vi "PathPlanner_PathConstraints_Test.vi"(8 "error in (no error)":errorcluster) -> (0 "error out":errorcluster, 3 "All Passed":bool)   [LabVIEW 2019]
uses:
  <vilib>/Rock Robotics/WPI/ThirdParty/JAS_Junk/TrajLib/Trajectory_Library.lvlib
  <vilib>/Rock Robotics/WPI/ThirdParty/MJansen/PathPlanner/PathPlanner24.lvlib
panel:
  out "Passed 2":bool
  out "Passed 1":bool
  # "Getters"
  # "JSON Parse"
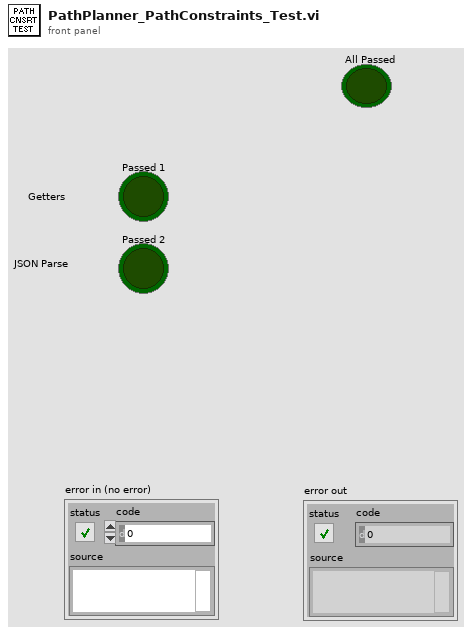
[diagram p1: front panel]
types:
  T1 = typedef "PathPlanner24.lvlib/PathPlannerPathConstraints.ctl" = cluster{"MaxVelocityMps;":dbl, "MaxAccelerationMpsSq;":dbl, "MaxAngularVelRadPsEc;":dbl, "MaxAngularAccRadPSecSq":dbl, "Exists":bool}
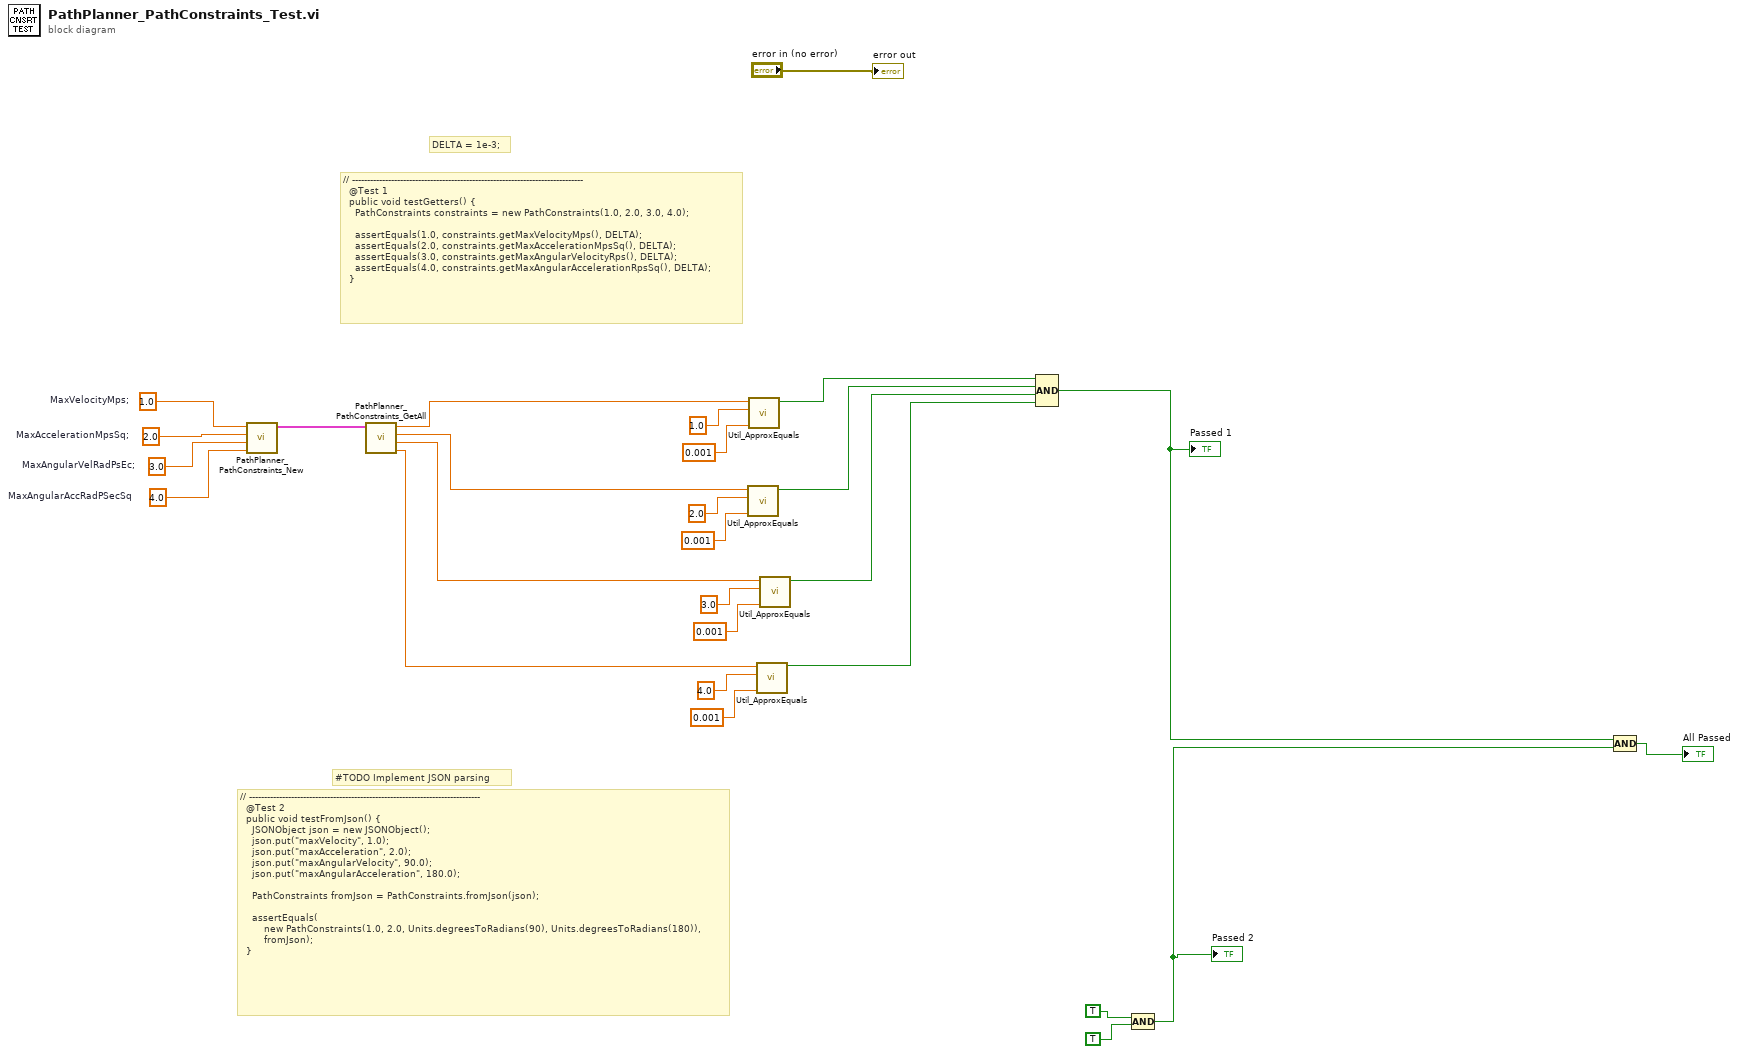
[diagram p0: block diagram]
diagram:
  w20 = 1.0  # MaxVelocityMps;
  w21 = 2.0  # MaxAccelerationMpsSq;
  w22 = 3.0  # MaxAngularVelRadPsEc;
  w23 = 4.0  # MaxAngularAccRadPSecSq
  # "#TODO Implement JSON parsing"
  # "// -----------------------------------------------------------------------------\n  @Test 2\n  public void testFromJson() {\n    JSONObject json = new JSONObject();\n    json.put(\"maxVelocity\", 1.0);\n    json.put(\"maxAcceleration\", 2.0);\n    json.put(\"maxAngularVelocity\", 90.0);\n    json.put(\"maxAngularAcceleration\", 180.0);\n\n    PathConstraints fromJson = PathConstraints.fromJson(json);\n\n    assertEquals(\n        new PathConstraints(1.0, 2.0, Units.degreesToRadians(90), Units.degreesToRadians(180)),\n        fromJson);\n  }"
  # "// -----------------------------------------------------------------------------\n  @Test 1\n  public void testGetters() {\n    PathConstraints constraints = new PathConstraints(1.0, 2.0, 3.0, 4.0);\n\n    assertEquals(1.0, constraints.getMaxVelocityMps(), DELTA);\n    assertEquals(2.0, constraints.getMaxAccelerationMpsSq(), DELTA);\n    assertEquals(3.0, constraints.getMaxAngularVelocityRps(), DELTA);\n    assertEquals(4.0, constraints.getMaxAngularAccelerationRpsSq(), DELTA);\n  }"
  # "DELTA = 1e-3;"
  n1 = call <vilib>:"PathPlanner_PathConstraints_New.vi"("MaxAngularAccRadPSecSq"=w23, "MaxAngularVelRadPsEc;"=w22, "MaxAccelerationMpsSq;"=w21, "MaxVelocityMps;"=w20) -> ("PathPlannerConstraints"=w14:T1)  [unwired: 7 in]
  n2 = call <vilib>:"PathPlanner_PathConstraints_GetAll.vi"("PathPlannerConstraints"=w14) -> ("MaxAngularAccRadPSecSq"=w6:dbl, "MaxAngularVelRadPsEc;"=w7:dbl, "MaxAccelerationMpsSq;"=w8:dbl, "MaxVelocityMps;"=w9:dbl)  [unwired: 7 in]
  n3 = call <vilib>:"Util_ApproxEquals.vi"("Tolerance"=0.001, "Value 2"=2.0, "Value 1"=w8) -> ("ApproxEquals"=w15:bool)  [unwired: 8 in]
  n4 = call <vilib>:"Util_ApproxEquals.vi"("Tolerance"=0.001, "Value 2"=1.0, "Value 1"=w9) -> ("ApproxEquals"=w25:bool)  [unwired: 8 in]
  n5 = call <vilib>:"Util_ApproxEquals.vi"("Tolerance"=0.001, "Value 2"=4.0, "Value 1"=w6) -> ("ApproxEquals"=w4:bool)  [unwired: 8 in]
  n6 = call <vilib>:"Util_ApproxEquals.vi"("Tolerance"=0.001, "Value 2"=3.0, "Value 1"=w7) -> ("ApproxEquals"=w5:bool)  [unwired: 8 in]
  n7 = Compound Arithmetic op=AND(w25, w15, w5, w4) -> (w24:bool)
  "Passed 1" <- w24
  n8 = Compound Arithmetic op=AND(TRUE, TRUE) -> (w1:bool)
  "Passed 2" <- w1
  n9 = Compound Arithmetic op=AND(w24, w1) -> (→"All Passed":bool)
  "error out" <- "error in (no error)"
